vi "副屏设置.vi"() -> ()   [LabVIEW 2016, in "副屏.lvlib"]
uses:
  <vilib>/Utility/config.llb/NI_LVConfig.lvlib
panel:
  in  "氟化物":bool caption="氨氮禁用"
  in  "ORP":bool caption="氨氮禁用"
  in  "启用副屏":bool=TRUE caption="氨氮禁用"
  in  "关闭":bool
  in  "底部状态栏显示信息":string="一体化微型水质监测系统"
  in  "流速":bool caption="氨氮禁用"
  in  "瞬时流量":bool caption="氨氮禁用"
  in  "湿度":bool=TRUE caption="氨氮禁用"
  in  "水位":bool caption="氨氮禁用"
  in  "室温":bool=TRUE caption="氨氮禁用"
  in  "CODCr":bool caption="氨氮禁用"
  in  "CODMn":bool caption="氨氮禁用"
  in  "总氮":bool caption="氨氮禁用"
  in  "总磷":bool caption="氨氮禁用"
  in  "氨氮":bool caption="氨氮禁用"
  in  "Turb":bool caption="氨氮禁用"
  in  "Cond":bool caption="氨氮禁用"
  in  "DO":bool caption="氨氮禁用"
  in  "pH":bool caption="氨氮禁用"
  in  "水温":bool caption="氨氮禁用"
  # "副屏显示信息设置"
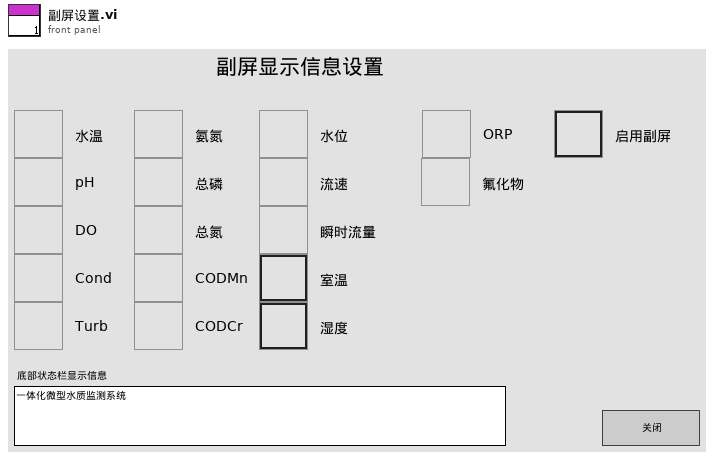
[diagram p1: front panel]
types:
  T1 = typedef "NI_LVConfig.lvlib/Config Data RefNum.ctl" = refnum<k1>
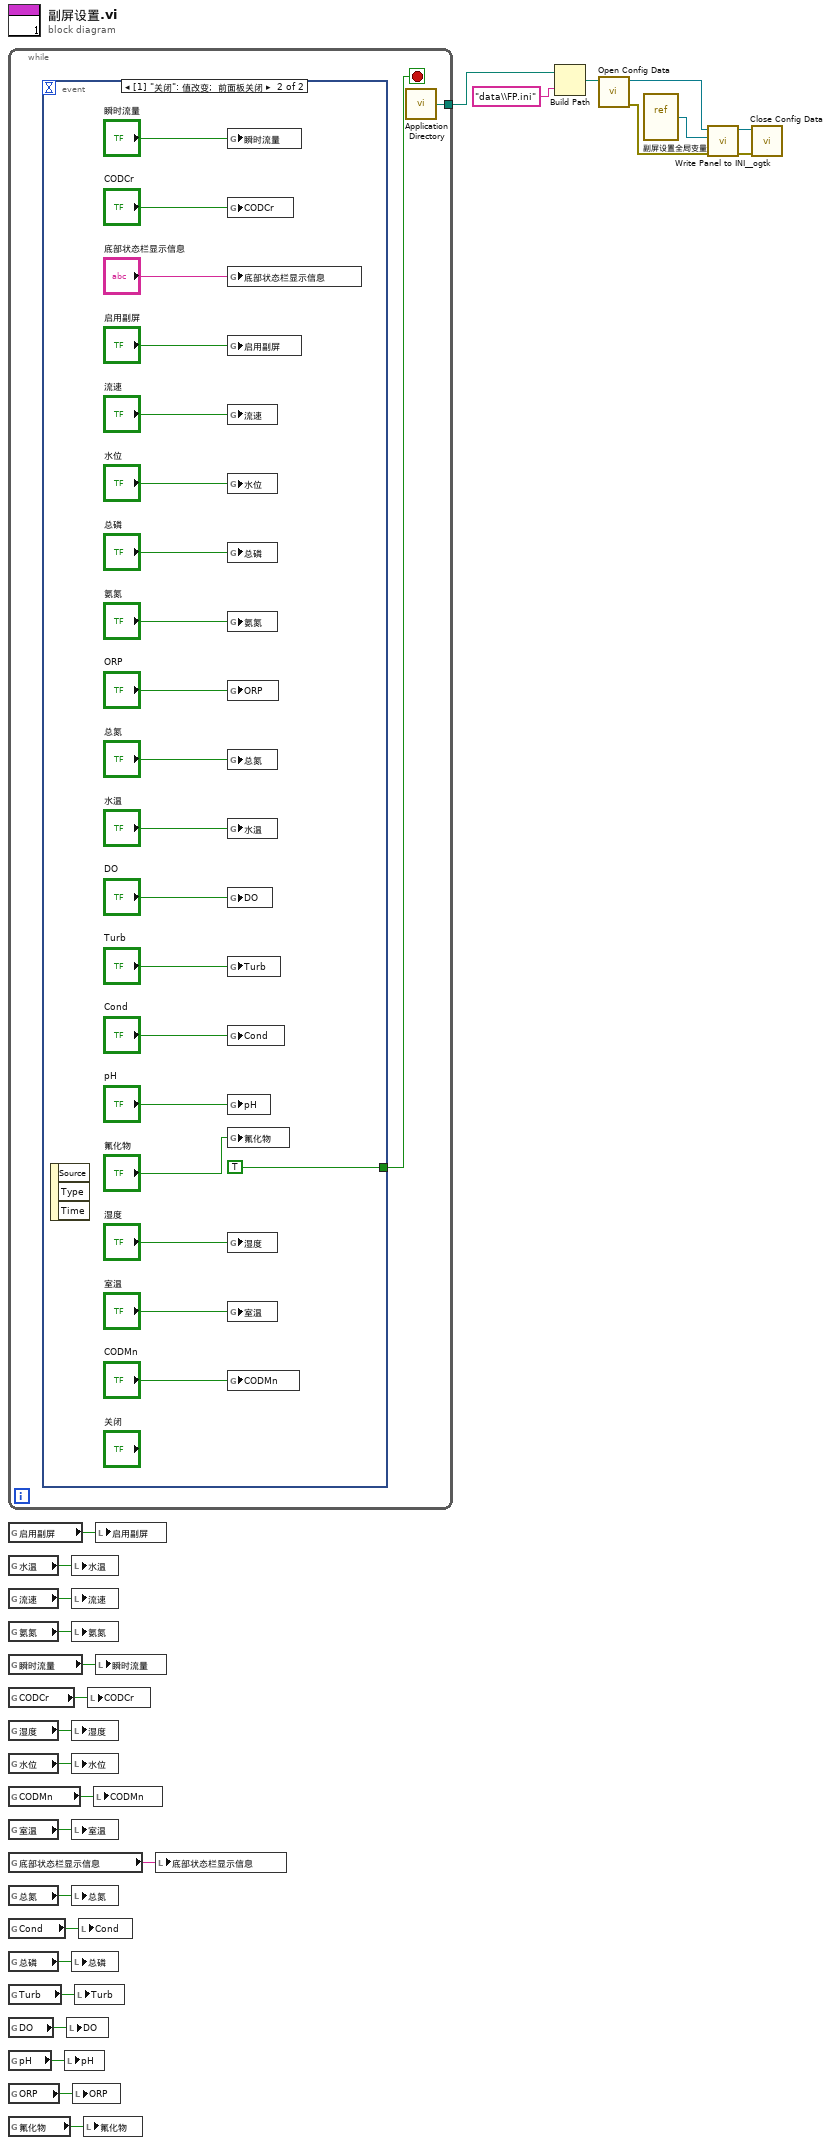
[diagram p0: block diagram]
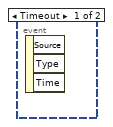
[diagram p2: hidden frame]
diagram:
  n1 = while {
    tunnel: [w28] -> w4
    stop <- w29 stop-if-true
    n2 = event shown="[1] \"关闭\": 值改变;  前面板关闭" {
      selector: _ -> [_ _]
      dyn-events: _ -> [_ _]
      timeout: _ -> [_ _]
      tunnel: [_ TRUE] -> w29
      event Timeout {
        n3 = event-data() -> ()  [unwired: 1 in, 3 out]
      }
      event "关闭": Value Change; Panel Close {
        n4 = event-data() -> ()  [unwired: 1 in, 3 out]
        n5 = global write "副屏设置全局变量.vi" "瞬时流量"("瞬时流量") -> ()
        n6 = global write "副屏设置全局变量.vi" "CODCr"("CODCr") -> ()
        n7 = global write "副屏设置全局变量.vi" "底部状态栏显示信息"("底部状态栏显示信息") -> ()
        n8 = global write "副屏设置全局变量.vi" "启用副屏"("启用副屏") -> ()
        n9 = global write "副屏设置全局变量.vi" "流速"("流速") -> ()
        n10 = global write "副屏设置全局变量.vi" "水位"("水位") -> ()
        n11 = global write "副屏设置全局变量.vi" "总磷"("总磷") -> ()
        n12 = global write "副屏设置全局变量.vi" "氨氮"("氨氮") -> ()
        n13 = global write "副屏设置全局变量.vi" "ORP"("ORP") -> ()
        n14 = global write "副屏设置全局变量.vi" "总氮"("总氮") -> ()
        n15 = global write "副屏设置全局变量.vi" "水温"("水温") -> ()
        n16 = global write "副屏设置全局变量.vi" "DO"("DO") -> ()
        n17 = global write "副屏设置全局变量.vi" "Turb"("Turb") -> ()
        n18 = global write "副屏设置全局变量.vi" "Cond"("Cond") -> ()
        n19 = global write "副屏设置全局变量.vi" "pH"("pH") -> ()
        n20 = global write "副屏设置全局变量.vi" "氟化物"("氟化物") -> ()
        n21 = global write "副屏设置全局变量.vi" "湿度"("湿度") -> ()
        n22 = global write "副屏设置全局变量.vi" "室温"("室温") -> ()
        n23 = global write "副屏设置全局变量.vi" "CODMn"("CODMn") -> ()
      }
    }
    n24 = call <vilib>:"Application Directory.vi"() -> ("Application Directory"=w28:path)
  }
  n25 = global read "副屏设置全局变量.vi" "启用副屏"() -> (w3:bool)
  n26 = global read "副屏设置全局变量.vi" "水温"() -> (w27:bool)
  n27 = global read "副屏设置全局变量.vi" "流速"() -> (w21:bool)
  n28 = global read "副屏设置全局变量.vi" "氨氮"() -> (w26:bool)
  n29 = global read "副屏设置全局变量.vi" "瞬时流量"() -> (w19:bool)
  n30 = global read "副屏设置全局变量.vi" "CODCr"() -> (w25:bool)
  n31 = global read "副屏设置全局变量.vi" "湿度"() -> (w18:bool)
  n32 = global read "副屏设置全局变量.vi" "水位"() -> (w24:bool)
  n33 = global read "副屏设置全局变量.vi" "CODMn"() -> (w23:bool)
  n34 = global read "副屏设置全局变量.vi" "室温"() -> (w15:bool)
  n35 = global read "副屏设置全局变量.vi" "底部状态栏显示信息"() -> (w22:string)
  n36 = global read "副屏设置全局变量.vi" "总氮"() -> (w16:bool)
  n37 = global read "副屏设置全局变量.vi" "Cond"() -> (w20:bool)
  n38 = global read "副屏设置全局变量.vi" "总磷"() -> (w13:bool)
  n39 = global read "副屏设置全局变量.vi" "Turb"() -> (w14:bool)
  n40 = global read "副屏设置全局变量.vi" "DO"() -> (w17:bool)
  n41 = global read "副屏设置全局变量.vi" "pH"() -> (w12:bool)
  n42 = global read "副屏设置全局变量.vi" "ORP"() -> (w2:bool)
  n43 = global read "副屏设置全局变量.vi" "氟化物"() -> (w1:bool)
  n44 = local write "pH"(w12) -> ()
  n45 = local write "DO"(w17) -> ()
  n46 = local write "水温"(w27) -> ()
  n47 = local write "流速"(w21) -> ()
  n48 = local write "氨氮"(w26) -> ()
  n49 = local write "湿度"(w18) -> ()
  n50 = local write "水位"(w24) -> ()
  n51 = local write "室温"(w15) -> ()
  n52 = local write "总氮"(w16) -> ()
  n53 = local write "总磷"(w13) -> ()
  n54 = local write "ORP"(w2) -> ()
  n55 = local write "Turb"(w14) -> ()
  n56 = local write "Cond"(w20) -> ()
  n57 = local write "氟化物"(w1) -> ()
  n58 = local write "CODCr"(w25) -> ()
  n59 = local write "CODMn"(w23) -> ()
  n60 = local write "启用副屏"(w3) -> ()
  n61 = local write "瞬时流量"(w19) -> ()
  n62 = local write "底部状态栏显示信息"(w22) -> ()
  n63 = Build Path(base path=w4, name or relative path="data\\FP.ini" ("名称或相对路径")) -> (appended path=w6:path)
  n64 = call <vilib>:"Open Config Data.vi"("configuration file path"=w6) -> ("error out"=w10:errorcluster, "refnum"=w7:T1)  [unwired: 8 in, 1 out]
  n65 = vi-ref "副屏设置全局变量.vi"() -> (w8:refnum<vi>)
  n66 = call <userlib>:"Write Panel to INI__ogtk.vi"("error in (no error)"=w10, "VI ref"=w8, "refnum"=w7) -> ("error out"=w11:errorcluster, "refnum out"=w9:T1)  [unwired: 7 in]
  n67 = call <vilib>:"Close Config Data.vi"("error in (no error)"=w11, "refnum"=w9) -> ()  [unwired: 8 in, 2 out]
